vi "write read until ts.vi"(4 "termination sequence (return)":string="\n", 5 "Max time (ms) (2000)":u32=2000, 6 "string to write":string, 7 "Port Number":refnum<visa-resource-name>) -> (0 "Time out":bool, 1 "return string":string, 2 "return code":string, 3 "command":string)   [LabVIEW 2012]
doc: "The Simple Serial VI performs a Serial Port read of the specified number of bytes. The VI polls the serial port until the number of bytes are available."
panel:
  # "PC:  0 = COM1, 1= COM2,...\nMac:  0 = Modem, 1 = Printer\nSun: 0 = ttya, 1 = ttyb,..."
  # "Read from Serial Port until termination sequence\n is found."
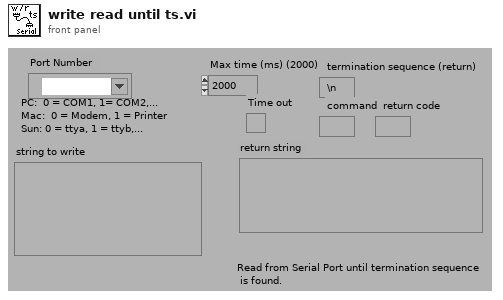
[diagram p1: front panel]
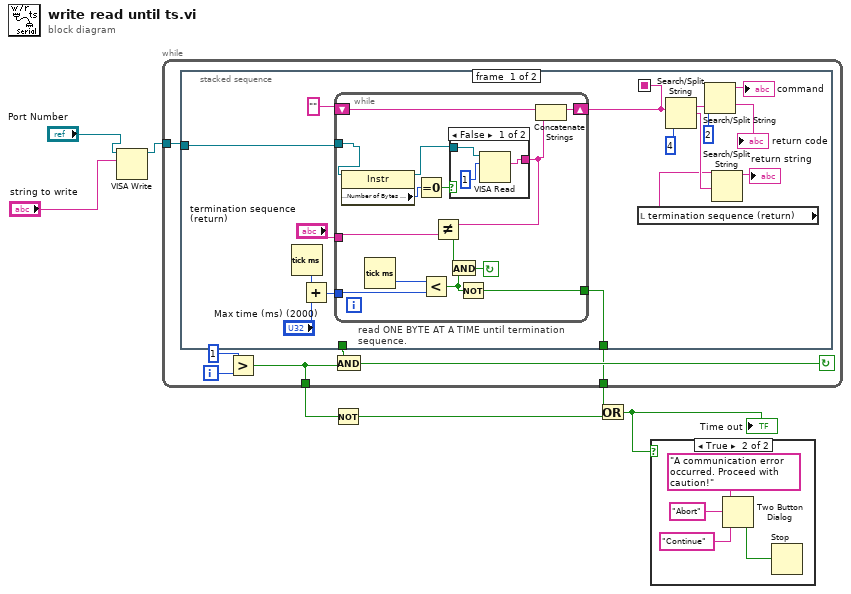
[diagram p0: block diagram]
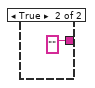
[diagram p2: hidden frame]
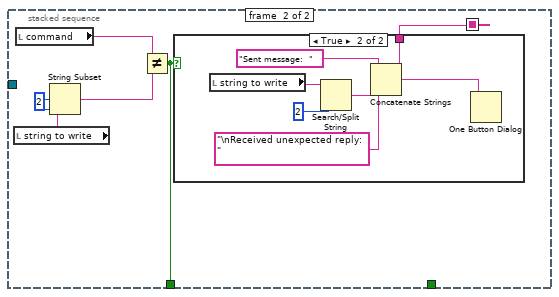
[diagram p3: hidden frame]
diagram:
  n1 = VISA Write(VISA resource name="Port Number", write buffer="string to write") -> (VISA resource name out=w1:refnum<visa-resource-name>)  [unwired: 1 in, 2 out]
  n2 = while {
    tunnel: [w8] -> w6
    tunnel: [w9] -> w7
    tunnel: w1 -> [w14]
    i -> [w11]
    stop <- w10 continue-if-true
    n3 = stacked-sequence {
      seq-local: [w19 _] -> [_ w54]
      tunnel: w14 -> [w21 _]
      tunnel: [_ w53] -> w13
      tunnel: [w15 _] -> w9
      frame #0 {
        n4 = Tick Count (ms)() -> (millisecond timer value=w23:u32)
        n5 = Add(x=w23, y="Max time (ms) (2000)") -> (x+y=w25:u32)
        n6 = while "read ONE BYTE AT A TIME until termination sequence." {
          shift-left: "" -> [w38]
          shift-right: [w37] -> w19
          tunnel: w25 -> [w42]
          tunnel: [w40] -> w15
          tunnel: "termination sequence (return)" -> [w35]
          tunnel: w21 -> [w32]
          stop <- w44 continue-if-true
          n7 = property class="Instr"(reference=w32) -> (reference out=w31:refnum<visa-resource-name>, "Serial Settings:Number of Bytes at Serial Port"=w33:u32)  [unwired: 1 in, 1 out]
          n8 = Tick Count (ms)() -> (millisecond timer value=w41:u32)
          n9 = Equal To 0?(x=w33) -> (x = 0?=w39:bool)
          n10 = Less?(x=w41, y=w42) -> (x < y?=w43:bool)
          n11 = case shown="False" w39 {
            tunnel: w31 -> [w46 _]
            tunnel: [w45 ""] -> w36
            frame False {
              n12 = VISA Read(VISA resource name=w46, byte count=1) -> (read buffer=w45:string)  [unwired: 1 in, 3 out]
            }
            frame True {
            }
          }
          n13 = Not Equal?(x=w36, y=w35) -> (x != y?=w34:bool)
          n14 = And(x=w34, y=w43) -> (x .and. y?=w44:bool)
          n15 = Not(x=w43) -> (.not. x?=w40:bool)
          n16 = Concatenate Strings(w38, w36) -> (w37:string)
        }
        n17 = local read "termination sequence (return)"() -> (w17:string)
        n18 = Search/Split String(string=w19, offset (0)=4) -> (substring before match=w27:string, match + rest of string=w18:string)  [unwired: 1 in, 1 out]
        n19 = Search/Split String(string=w27, offset (0)=2) -> (substring before match=→"command":string, match + rest of string=→"return code":string)  [unwired: 1 in, 1 out]
        n20 = Search/Split String(string=w18, search string/char (-)=w17) -> (substring before match=→"return string":string)  [unwired: 1 in, 2 out]
      }
      frame #1 {
        w51 = 2
        n21 = local read "string to write"() -> (w52:string)
        n22 = local read "command"() -> (w50:string)
        n23 = String Subset(string=w52, offset (0)=w51, length (rest)=w51) -> (substring=w49:string)
        n24 = Not Equal?(x=w50, y=w49) -> (x != y?=w53:bool)
        n25 = case shown="True" w53 {
          tunnel: w54 -> [_ w60]
          frame False {
          }
          frame True {
            n26 = local read "string to write"() -> (w58:string)
            n27 = Search/Split String(string=w58, offset (0)=2) -> (match + rest of string=w56:string)  [unwired: 1 in, 2 out]
            n28 = Concatenate Strings("Sent message:  ", w56, "\nReceived unexpected reply:  ", w60) -> (w61:string)
            n29 = One Button Dialog(message=w61) -> ()  [unwired: 1 in, 1 out]
          }
        }
      }
    }
    n30 = Greater?(x=1, y=w11) -> (0:w8:bool)
    n31 = And(x=w13, y=w8) -> (x .and. y?=w10:bool)
  }
  n32 = Not(x=w6) -> (.not. x?=w5:bool)
  n33 = Or(x=w7, y=w5) -> (x .or. y?=w4:bool)
  "Time out" <- w4
  n34 = case shown="True" w4 {
    frame False {
    }
    frame True {
      n35 = Two Button Dialog(message="A communication error occurred. Proceed with caution!", 1:"Continue", 2:"Abort") -> (T button?=w62:bool)
      n36 = Stop(stop? (T)=w62) -> ()
    }
  }
